vi "Side_Vertical_Lancing_Integrated.vi"(0 "Image Out":T1(plugin-control), 1 "Ref ROI Search Direction":u32(ring)=2 items=["Left to Right", "Right to Left", "Top to Bottom", "Bottom to Top"], 2 "Ref ROI Edge Options":T4={"Edge Polarity"=2, "Kernel Size"=3, "Width"=3, "Minimum Edge Strength"=50.0, "Interpolation Type"=enum."Zero Order", "Data Processing Method"=enum."Average"} {"Edge Polarity" items=["All Edges", "Rising Edges", "Falling Edges"]; "Minimum Edge Strength" format="%.2f"; "Width" step=2; "Kernel Size" step=2}, 3 "Ref ROI Line Options":T7={"Number of Lines"=1, "Type"=enum."First Edge Rake", "Min. Score"=10.0, "Max. Score"=1000.0, "Orientation"=4.0, "Angle Range"=40.0, "Angle Tolerance"=4.0, "Step Size"=8, "Min. SNR (db)"=0.0, "Min. Points (%)"=25.0, "Hough Iterations"=5} {"Min. Points (%)" min=0.0 max=100.0; "Min. SNR (db)" min=0.0; "Max. Score" min=0.0 max=1024.0; "Min. Score" min=0.0 max=1024.0 step=1.0}, 4 "ROI 1 Edge Options":T4={"Edge Polarity"=2, "Kernel Size"=3, "Width"=3, "Minimum Edge Strength"=50.0, "Interpolation Type"=enum."Bilinear Fixed", "Data Processing Method"=enum."Average"} {"Edge Polarity" items=["All Edges", "Rising Edges", "Falling Edges"]; "Minimum Edge Strength" format="%.2f"; "Width" step=2; "Kernel Size" step=2}, 5 "ROI 1 Step Size":u32=5, 6 "ROI 1 Process":T6(ring)=enum."Get Best Edge", 7 "error in (no error)":errorcluster, 8 "Calibrated Image":T1, 9 "ROI 1 Scan Direction":u16(ring)=3 items=["Left To Right", "Right To Left", "Top To Bottom", "Bottom To Top"], 10 "Ref ROI After SV Transformation":T3 {"Contours"."Type" items=["No Selection", "Point", "Line", "Rectangle", "Oval", "Polygon", "Free", "Annulus", "Unused2", "Unused3", "Broken Line", "Free Hand Line", "Rotated Rectangle"]}, 11 "Measurement ROI 1 Before Tranformation":T3 {"Contours"."Type" items=["No Selection", "Point", "Line", "Rectangle", "Oval", "Polygon", "Free", "Annulus", "Unused2", "Unused3", "Broken Line", "Free Hand Line", "Rotated Rectangle"]}, 12 "Ellipse Center":cluster{"Center X":dbl, "Center Y":dbl}) -> (18 "Overlay Arrow Lines":T2, 20 "Measurement Lancing":sgl, 27 "error out":errorcluster)   [LabVIEW 2019, in "Algorithm.lvclass"]
uses:
  FrameworkOverrides/Algorithm.lvclass
  <vilib>/vision/NI_Vision_Development_Module.lvlib
  <vilib>/vision/Measure.llb/Edge Polarity.ctl
  <vilib>/vision/Measure.llb/Edge Options.ctl
  <vilib>/vision/Measure.llb/Straight Edge Process.ctl
  <vilib>/vision/Measure.llb/Straight Edge Options.ctl
  <vilib>/vision/Image Controls.llb/IMAQ Image.ctl
panel:
  out "Distance":dbl format="%.2f"
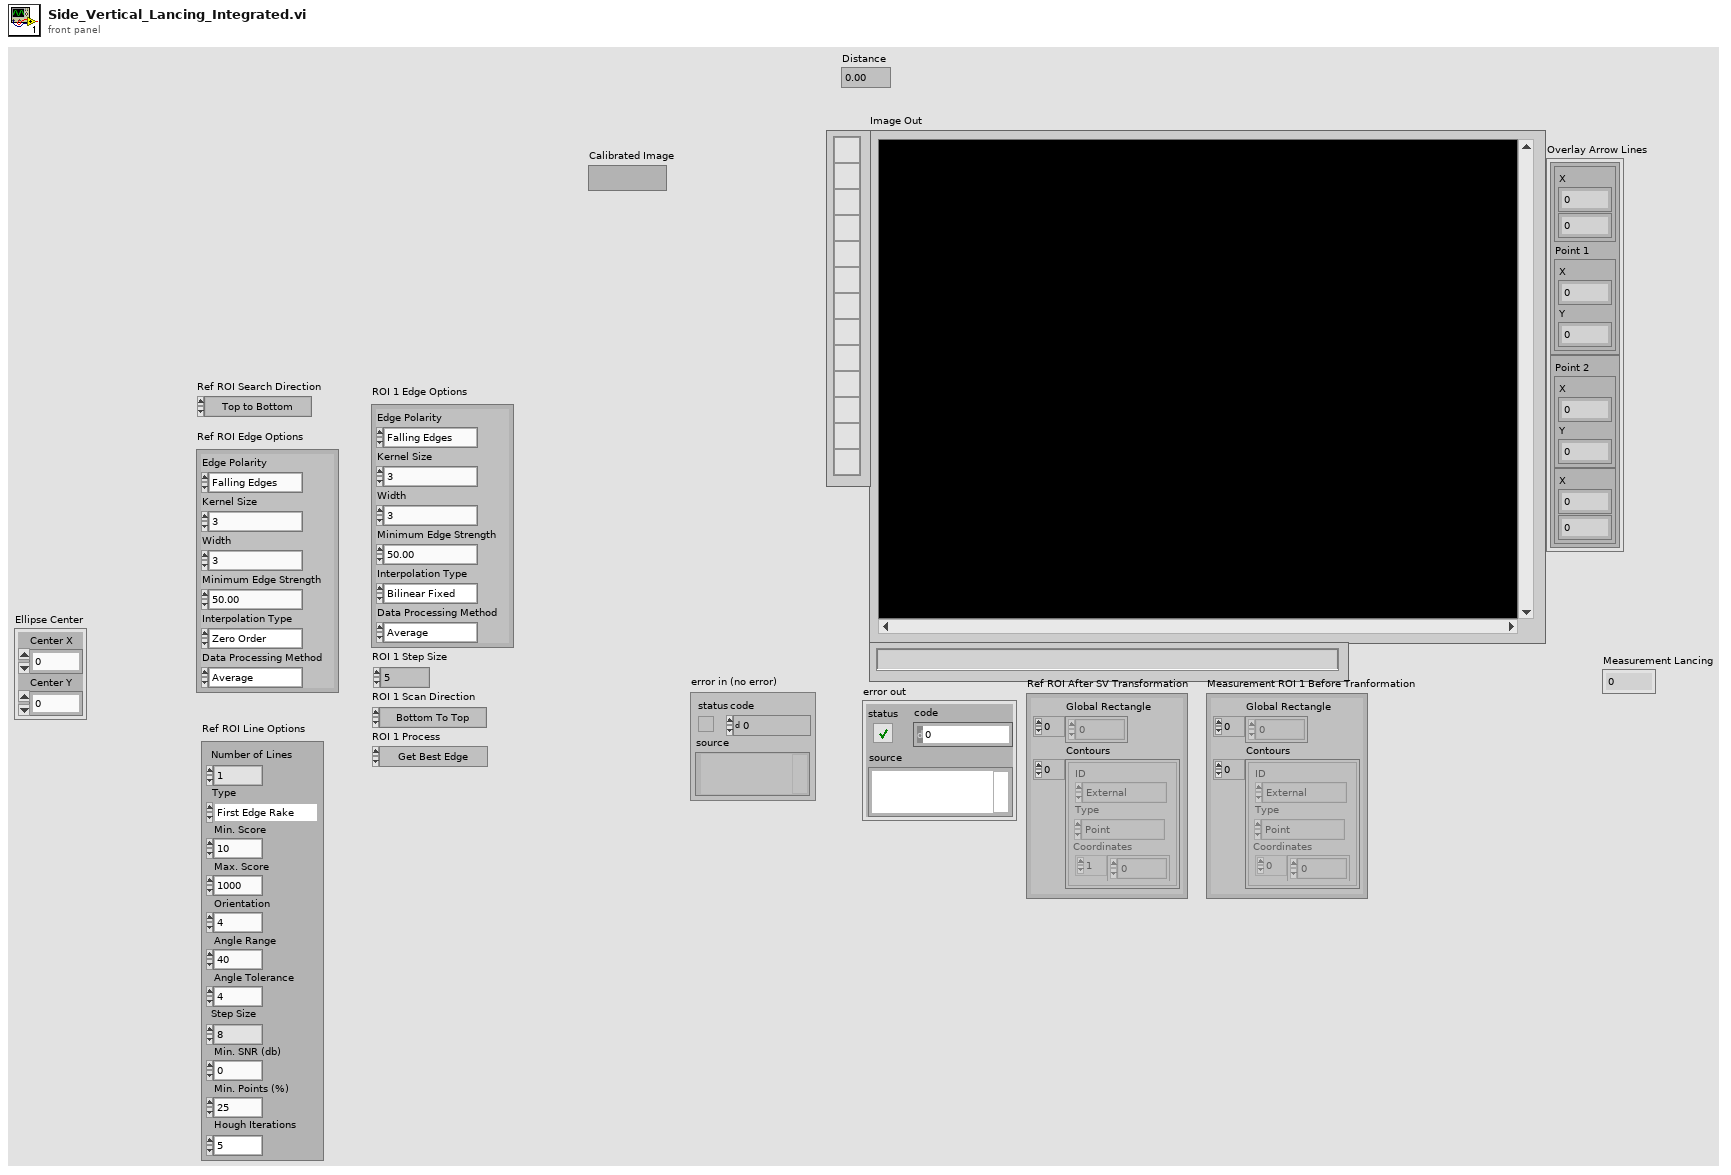
[diagram p1: front panel]
types:
  T1 = typedef "IMAQ Image.ctl" = refnum<image>
  T2 = cluster{cluster{cluster{"X":sgl, sgl}, "Point 1":cluster{"X":sgl, "Y":sgl}}, cluster{"Point 2":cluster{"X":sgl, "Y":sgl}, cluster{"X":sgl, sgl}}}
  T3 = cluster{"Global Rectangle":i32[], "Contours":cluster{"ID":enum32{"External", "Internal"}, "Type":u32, "Coordinates":i32[]}[]}
  T4 = typedef "Edge Options.ctl" = cluster{"Edge Polarity":T5, "Kernel Size":u32, "Width":u32, "Minimum Edge Strength":sgl, "Interpolation Type":enum32{"Zero Order", "Bilinear", "Quadratic", "Cubic", "Bilinear Fixed"}, "Data Processing Method":enum32{"Average", "Median"}}
  T5 = typedef "Edge Polarity.ctl" = u32
  T6 = enum16{"Get First Edge", "Get First + Last Edge", "Get All Edges", "Get Best Edge"}
  T7 = typedef "Straight Edge Options.ctl" = cluster{"Number of Lines":i32, "Type":T8, "Min. Score":dbl, "Max. Score":dbl, "Orientation":dbl, "Angle Range":dbl, "Angle Tolerance":dbl, "Step Size":u32, "Min. SNR (db)":dbl, "Min. Points (%)":dbl, "Hough Iterations":i32}
  T8 = typedef "Straight Edge Process.ctl" = enum32{"First Edge Rake", "Best Edge Rake", "Hough Edge Rake", "First Edge Projection", "Best Edge Projection"}
  T9 = cluster{"Point 1":cluster{"X":sgl, "Y":sgl}, "Point 2":cluster{"X":sgl, "Y":sgl}}
  T10 = cluster{"Point1 (Pixels)":cluster{"X":sgl, "Y":sgl}, "Point2 (Pixels)":cluster{"X":sgl, "Y":sgl}, "Point1 (Real-World)":cluster{"X":sgl, "Y":sgl}, "Point2 (Real-World)":cluster{"X":sgl, "Y":sgl}, "Angle (Pixel)":dbl, "Angle (Real-World)":dbl, "Score":dbl, "Straightness":dbl, "Average SNR (db)":dbl, "Calibration Valid":bool}[]
  T11 = cluster{"Left":dbl, "Top":dbl, "Right":dbl, "Bottom":dbl, "Angle":dbl}
  T12 = typedef "ROI Descriptor" = cluster{"Global Rectangle":i32[], "Contours":cluster{"ID":enum32{"External", "Internal"}, "Type":u32, "Coordinates":i32[]}[]}
  T13 = typedef "Edge New.ctl" = cluster{"Location (Pixel)":cluster{"X":sgl, "Y":sgl}, "Location (Real-World)":cluster{"X":sgl, "Y":sgl}, "Distance (Pixel)":dbl, "Distance (Real-World)":dbl, "Strength":dbl, "Noise":dbl, "Rising?":bool}
  T14 = cluster{"Point1 (Pixels)":cluster{"X":sgl, "Y":sgl}, "Point2 (Pixels)":cluster{"X":sgl, "Y":sgl}, "Point1 (Real-World)":cluster{"X":sgl, "Y":sgl}, "Point2 (Real-World)":cluster{"X":sgl, "Y":sgl}, "Angle (Pixel)":dbl, "Angle (Real-World)":dbl, "Score":dbl, "Straightness":dbl, "Average SNR (db)":dbl, "Calibration Valid":bool}
  T15 = cluster{cluster{"X":sgl, sgl}, "Point 1":cluster{"X":sgl, "Y":sgl}}
  T16 = cluster{"Point 2":cluster{"X":sgl, "Y":sgl}, cluster{"X":sgl, sgl}}
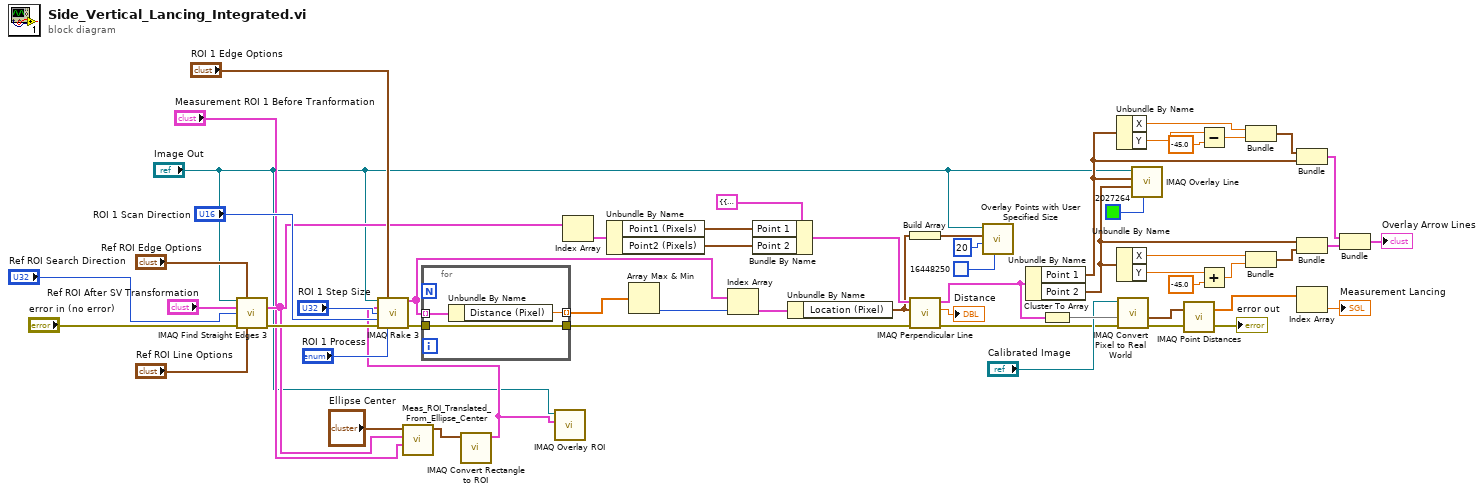
[diagram p0: block diagram]
diagram:
  n1 = call "IMAQ Find Straight Edges 3"("Image"="Image Out", "Edge Options"="Ref ROI Edge Options", "ROI Descriptor"="Ref ROI After SV Transformation", "Search Direction"="Ref ROI Search Direction", "error in (no error)"="error in (no error)", "Line Options"="Ref ROI Line Options") -> ("Straight Edges"=w5:T10, "error out"=w53:errorcluster)  [unwired: 5 in, 3 out]
  n2 = call "Meas_ROI_Translated_From_Ellipse_Center.vi"("ROI Descriptor"="Measurement ROI 1 Before Tranformation", "Straight Edges"=w5, "Ellipse Center"="Ellipse Center") -> ("Translated ROI"=w3:T11)  [unwired: 8 in]
  n3 = call "IMAQ Convert Rectangle to ROI"("Rectangle"=w3) -> ("ROI Descriptor"=w2:T12)  [unwired: 8 in, 1 out]
  n4 = call "IMAQ Rake 3"("Image"="Image Out", "Edge Options"="ROI 1 Edge Options", "ROI Descriptor"=w2, "Step Size"="ROI 1 Step Size", "Scan Direction"="ROI 1 Scan Direction", "error in (no error)"=w53, "Process"="ROI 1 Process") -> ("First Edges"=w47:T13[], "error out"=w46:errorcluster)  [unwired: 5 in, 2 out]
  n5 = for {
    tunnel: w47 -> [w60] mode=indexing
    tunnel: [w59] -> w49 mode=indexing
    tunnel: w46 -> [w58]
    tunnel: [w58] -> w38
    n6 = Unbundle By Name(w60) -> ("Distance (Pixel)"=w59:dbl)
  }
  n7 = call "IMAQ Overlay ROI"("ROI Descriptor"=w2, "Image"="Image Out") -> ()  [unwired: 8 in, 2 out]
  n8 = Index Array(array=w5) -> (element=w43:T14)  [unwired: 1 in]
  n9 = Unbundle By Name(w43) -> ("Point1 (Pixels)"=w41:cluster{"X":sgl, "Y":sgl}, "Point2 (Pixels)"=w40:cluster{"X":sgl, "Y":sgl})
  n10 = Array Max & Min(array=w49) -> (min index (indices)=w48:i32)  [unwired: 3 out]
  n11 = Index Array(array=w47, index=w48) -> (element=w44:T13)
  n12 = Bundle By Name(cluster=T9 {"Point 1"={"X"=0.0, "Y"=0.0}, "Point 2"={"X"=0.0, "Y"=0.0}} ("Line"), "Point 1"=w41, "Point 2"=w40) -> (w39:T9)
  n13 = Unbundle By Name(w44) -> ("Location (Pixel)"=w37:cluster{"X":sgl, "Y":sgl})
  n14 = Build Array(w37) -> (w36:cluster{"X":sgl, "Y":sgl}[])
  n15 = call "IMAQ Perpendicular Line"("error in (no error)"=w38, "Point"=w37, "Line"=w39) -> ("error out"=w12:errorcluster, "Distance"=→"Distance":dbl, "Perpendicular Line"=w15:T9)  [unwired: 6 in]
  n16 = call "Overlay Points with User Specified Size.vi"("Color"=u32 16448250, "Point Diameter (5)"=u32 20, "Points"=w36, "Image In"="Image Out") -> ()  [unwired: 6 in, 2 out]
  n17 = Unbundle By Name(w15) -> ("Point 1"=w30:cluster{"X":sgl, "Y":sgl}, "Point 2"=w29:cluster{"X":sgl, "Y":sgl})
  n18 = Cluster To Array(cluster=w15) -> (array=w14:cluster{"X":sgl, "Y":sgl}[])
  n19 = Unbundle By Name(w30) -> ("X"=w21:sgl, "Y"=w22:sgl)
  n20 = Unbundle By Name(w29) -> ("X"=w26:sgl, "Y"=w28:sgl)
  n21 = call "IMAQ Convert Pixel to Real World"("error in (no error)"=w12, "Array of Pixel Coordinates"=w14, "Calibrated Image"="Calibrated Image") -> ("error out"=w11:errorcluster, "Array of Real World Coordinates"=w10:cluster{"X":sgl, "Y":sgl}[])  [unwired: 3 in, 4 out]
  n22 = call "IMAQ Overlay Line"("Color"=u32 2027264, "End Point"=w29, "Start Point"=w30, "Image"="Image Out") -> ()  [unwired: 6 in, 2 out]
  n23 = call "IMAQ Point Distances"("Points"=w10, "error in (no error)"=w11) -> ("Distances"=w9:sgl[], "error out"=→"error out":errorcluster)  [unwired: 3 in]
  n24 = Subtract(x=w22, y=sgl -45.0) -> (x-y=w20:sgl)
  n25 = Add(x=w28, y=sgl -45.0) -> (x+y=w25:sgl)
  n26 = Bundle("X"=w21, w20) -> (w19:cluster{"X":sgl, sgl})  [unwired: 1 in]
  n27 = Bundle("X"=w26, w25) -> (w24:cluster{"X":sgl, sgl})  [unwired: 1 in]
  n28 = Bundle(w19, "Point 1"=w30) -> (w18:T15)  [unwired: 1 in]
  n29 = Bundle("Point 2"=w29, w24) -> (w17:T16)  [unwired: 1 in]
  n30 = Index Array(array=w9) -> (element=→"Measurement Lancing":sgl)  [unwired: 1 in]
  n31 = Bundle(w18, w17) -> (→"Overlay Arrow Lines":T2)  [unwired: 1 in]
